vi "KlingerV2 GetAxisParams.vi"(0 "Axe":u8(ring) items=["W", "X", "Y", "Z"], 5 "Param":T1, 11 "error in":errorcluster) -> (1 "ID Number":i32, 2 "Speed":cluster{"Vitesse":i32, "Accel":dbl}={"Vitesse"=800, "Accel"=0.4000000059604645} {"Accel" min=0.10000000149011612 max=2.0 step=0.10000000149011612 format="%#.1f"; "Vitesse" min=32 max=4000 step=1 format="%#.0f"}, 3 "TypeMouv":i32(ring) caption="Type de mouvement" items=["Linéaire", "Rotation"], 4 "Nom de l'axe":string, 6 "Type":i32(ring) caption="Type de moteur" items=["UE30", "UE72"], 8 "FactConv":dbl=0.01 caption="Facteur de\nConversion\n(m/pas ou °/pas)", 10 "CorrParams":T2={"CorrActive"=FALSE, "ErreurLim"=0.1, "NbrEssais"=3} caption="Paramètres de correction de position" {"NbrEssais" min=1 max=5 step=1; "ErreurLim" min=0.0 max=10.0 step=0.1 format="%#.1f"}, 13 "Encodeur":bool caption="Possède un\nEncodeur", 14 "Origine":bool caption="Possède un\nInterrupteur d'origine", 15 "error out":errorcluster)   [LabVIEW 2010]
doc: "Ce Vi lit les paramètres des différents axes moteur, qui sont enregistrer dans un fichier .ini."
uses:
  <userlib>/KlingerV2/KlingerV2 Params.ctl
  <vilib>/Utility/config.llb/Read Key (I32).vi
  <vilib>/Utility/config.llb/Read Key (Double).vi
  <vilib>/Utility/config.llb/Read Key (Boolean).vi
  <vilib>/Utility/config.llb/Read Key (String).vi
  <vilib>/Utility/config.llb/NI_LVConfig.lvlib
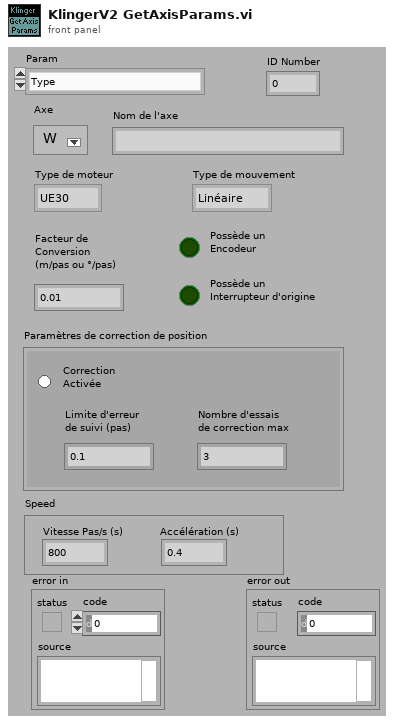
[diagram p1: front panel]
types:
  T1 = typedef "KlingerV2 Params.ctl" = enum16{"Type", "Origine", "Encodeur", "TypeMouv", "FactConv", "Nom", "CorrParams", "KlingCtrlPar", "Speed", "Acc", "Avance", "Tous"}
  T2 = cluster{"CorrActive":bool, "ErreurLim":dbl, "NbrEssais":i32}
  T3 = typedef "NI_LVConfig.lvlib/Config Data RefNum.ctl" = refnum<k1>
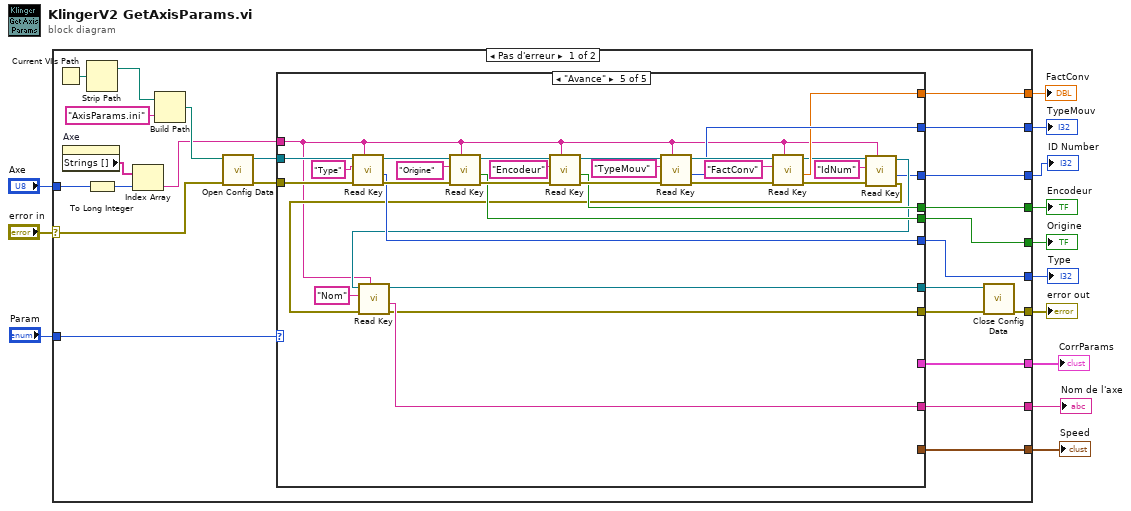
[diagram p0: block diagram]
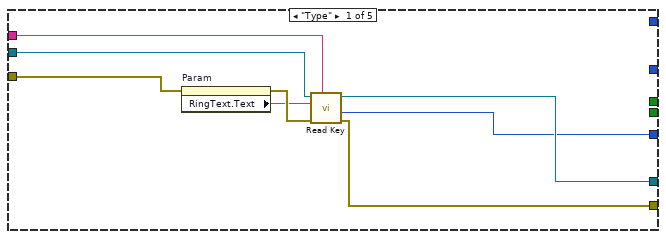
[diagram p2: hidden frame]
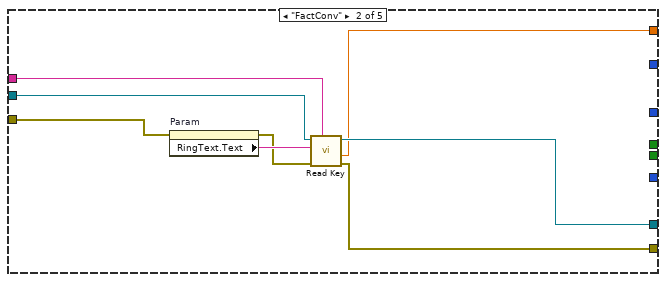
[diagram p3: hidden frame]
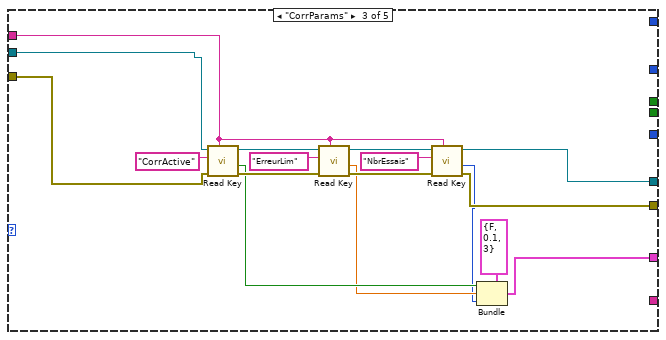
[diagram p4: hidden frame]
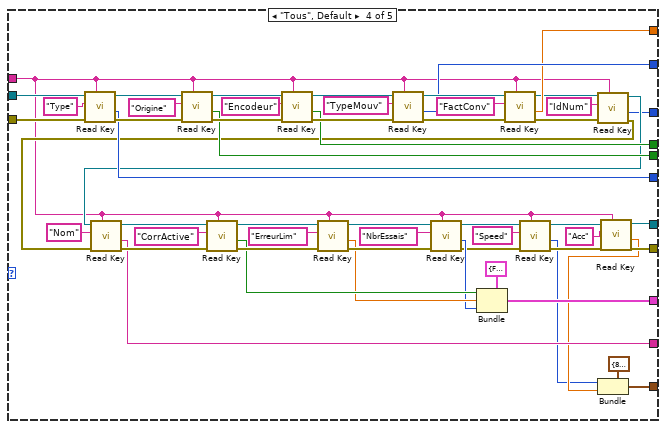
[diagram p5: hidden frame]
diagram:
  n1 = case shown="Pas d'erreur" "error in" {
    selector: "error in" -> [w34 w156]
    tunnel: "Axe" -> [w33 _]
    tunnel: [w26 w156] -> w12
    tunnel: [w23 _] -> w10
    tunnel: [w22 _] -> w9
    tunnel: [w21 _] -> w8
    tunnel: [w20 _] -> w7
    tunnel: [w19 _] -> w6
    tunnel: [w18 _] -> w5
    tunnel: [w17 _] -> w4
    tunnel: "Param" -> [w16 _]
    tunnel: [w15 _] -> w2
    tunnel: [w14 _] -> w1
    frame No Error {
      n2 = Current VI's Path() -> (path=w37:path)
      n3 = property on="Axe" class="MDér (strict)"() -> ("Strings []"=w31:string[])  [unwired: 2 in, 2 out]
      n4 = Strip Path(path=w37) -> (stripped path=w24:path)  [unwired: 1 out]
      n5 = To Long Integer(number=w33) -> (32bit integer=w32:i32)
      n6 = Index Array(array=w31, index=w32) -> (element=w25:string)
      n7 = Build Path(base path=w24, name or relative path="AxisParams.ini") -> (appended path=w35:path)
      n8 = call <vilib>:"Open Config Data.vi"("error in (no error)"=w34, "configuration file path"=w35) -> ("error out"=w29:errorcluster, "refnum"=w30:T3)  [unwired: 7 in, 1 out]
      n9 = case shown="\"Avance\"" w16 {
        tunnel: w30 -> [w45 w53 w61 w116 w150]
        tunnel: w29 -> [w40 w47 w59 w115 w149]
        tunnel: [w42 w50 w60 w84 w126] -> w28
        tunnel: [w43 w51 w63 w87 w125] -> w27
        tunnel: w25 -> [w44 w52 w62 w71 w127]
        tunnel: [_ w49 _ w77 w133] -> w23
        tunnel: [_ _ _ w95 w139] -> w22
        tunnel: [_ _ _ w94 w138] -> w21
        tunnel: [_ _ _ w93 w137] -> w20
        tunnel: [w41 _ _ w92 w136] -> w19
        tunnel: [_ _ w54 w91 _] -> w18
        tunnel: [_ _ _ w90 w135] -> w17
        tunnel: [_ _ _ w79 _] -> w15
        tunnel: [_ _ _ w72 w128] -> w14
        frame "Type" {
          n10 = property on="Param" class="Énum (strict)"(error in=w40) -> (error out=w39:errorcluster, "RingText.Text"=w38:string)  [unwired: 1 in, 1 out]
          n11 = call-poly <vilib>:"Read Key.vi"("section"=w44, "error in (no error)"=w39, "key"=w38, "refnum"=w45) -> ("error out"=w43:errorcluster, "value"=w41:i32, "refnum out"=w42:T3)  [unwired: 4 in, 1 out]
        }
        frame "FactConv" {
          n12 = property on="Param" class="Énum (strict)"(error in=w47) -> (error out=w46:errorcluster, "RingText.Text"=w48:string)  [unwired: 1 in, 1 out]
          n13 = call-poly <vilib>:"Read Key.vi"("section"=w52, "error in (no error)"=w46, "key"=w48, "refnum"=w53) -> ("error out"=w51:errorcluster, "value"=w49:dbl, "refnum out"=w50:T3)  [unwired: 4 in, 1 out]
        }
        frame "CorrParams" {
          n14 = call-poly <vilib>:"Read Key.vi"("section"=w62, "error in (no error)"=w59, "key"="CorrActive", "refnum"=w61) -> ("error out"=w66:errorcluster, "value"=w57:bool, "refnum out"=w67:T3)  [unwired: 4 in, 1 out]
          n15 = call-poly <vilib>:"Read Key.vi"("section"=w62, "error in (no error)"=w66, "key"="ErreurLim", "refnum"=w67) -> ("error out"=w64:errorcluster, "value"=w56:dbl, "refnum out"=w65:T3)  [unwired: 4 in, 1 out]
          n16 = call-poly <vilib>:"Read Key.vi"("section"=w62, "error in (no error)"=w64, "key"="NbrEssais", "refnum"=w65) -> ("error out"=w63:errorcluster, "value"=w55:i32, "refnum out"=w60:T3)  [unwired: 4 in, 1 out]
          n17 = Bundle(cluster=T2 {"CorrActive"=FALSE, "ErreurLim"=0.1, "NbrEssais"=3} ("CorrParams"), "CorrActive"=w57, "ErreurLim"=w56, "NbrEssais"=w55) -> (w54:T2)
        }
        frame "Tous", Default {
          n18 = call-poly <vilib>:"Read Key.vi"("section"=w71, "error in (no error)"=w115, "key"="Type", "refnum"=w116) -> ("error out"=w112:errorcluster, "value"=w92:i32, "refnum out"=w114:T3)  [unwired: 4 in, 1 out]
          n19 = call-poly <vilib>:"Read Key.vi"("section"=w71, "error in (no error)"=w112, "key"="Origine", "refnum"=w114) -> ("error out"=w111:errorcluster, "value"=w93:bool, "refnum out"=w106:T3)  [unwired: 4 in, 1 out]
          n20 = call-poly <vilib>:"Read Key.vi"("section"=w71, "error in (no error)"=w111, "key"="Encodeur", "refnum"=w106) -> ("error out"=w110:errorcluster, "value"=w94:bool, "refnum out"=w107:T3)  [unwired: 4 in, 1 out]
          n21 = call-poly <vilib>:"Read Key.vi"("section"=w71, "error in (no error)"=w110, "key"="TypeMouv", "refnum"=w107) -> ("error out"=w109:errorcluster, "value"=w95:i32, "refnum out"=w108:T3)  [unwired: 4 in, 1 out]
          n22 = call-poly <vilib>:"Read Key.vi"("section"=w71, "error in (no error)"=w109, "key"="FactConv", "refnum"=w108) -> ("error out"=w78:errorcluster, "value"=w77:dbl, "refnum out"=w76:T3)  [unwired: 4 in, 1 out]
          n23 = call-poly <vilib>:"Read Key.vi"("section"=w71, "error in (no error)"=w78, "key"="IdNum", "refnum"=w76) -> ("error out"=w74:errorcluster, "value"=w72:i32, "refnum out"=w75:T3)  [unwired: 4 in, 1 out]
          n24 = call-poly <vilib>:"Read Key.vi"("section"=w71, "error in (no error)"=w74, "key"="Nom", "refnum"=w75) -> ("error out"=w104:errorcluster, "value"=w90:string, "refnum out"=w105:T3)  [unwired: 4 in, 1 out]
          n25 = call-poly <vilib>:"Read Key.vi"("section"=w71, "error in (no error)"=w104, "key"="CorrActive", "refnum"=w105) -> ("error out"=w102:errorcluster, "value"=w98:bool, "refnum out"=w103:T3)  [unwired: 4 in, 1 out]
          n26 = call-poly <vilib>:"Read Key.vi"("section"=w71, "error in (no error)"=w102, "key"="ErreurLim", "refnum"=w103) -> ("error out"=w100:errorcluster, "value"=w97:dbl, "refnum out"=w101:T3)  [unwired: 4 in, 1 out]
          n27 = call-poly <vilib>:"Read Key.vi"("section"=w71, "error in (no error)"=w100, "key"="NbrEssais", "refnum"=w101) -> ("error out"=w88:errorcluster, "value"=w96:i32, "refnum out"=w89:T3)  [unwired: 4 in, 1 out]
          n28 = Bundle(cluster=T2 {"CorrActive"=FALSE, "ErreurLim"=0.1, "NbrEssais"=3} ("CorrParams"), "CorrActive"=w98, "ErreurLim"=w97, "NbrEssais"=w96) -> (w91:T2)
          n29 = call-poly <vilib>:"Read Key.vi"("section"=w71, "error in (no error)"=w88, "key"="Speed", "refnum"=w89) -> ("error out"=w87:errorcluster, "value"=w80:i32, "refnum out"=w85:T3)  [unwired: 4 in, 1 out]
          n30 = call-poly <vilib>:"Read Key.vi"("section"=w71, "key"="Acc", "refnum"=w85) -> ("value"=w81:dbl, "refnum out"=w84:T3)  [unwired: 5 in, 2 out]
          n31 = Bundle(cluster=cluster{"Vitesse":i32, "Accel":dbl} {"Vitesse"=800, "Accel"=0.4000000059604645} ("Speed"), "Vitesse"=w80, "Accel"=w81) -> (w79:cluster{"Vitesse":i32, "Accel":dbl})
        }
        frame "Avance" {
          n32 = call-poly <vilib>:"Read Key.vi"("section"=w127, "error in (no error)"=w149, "key"="Type", "refnum"=w150) -> ("error out"=w146:errorcluster, "value"=w136:i32, "refnum out"=w148:T3)  [unwired: 4 in, 1 out]
          n33 = call-poly <vilib>:"Read Key.vi"("section"=w127, "error in (no error)"=w146, "key"="Origine", "refnum"=w148) -> ("error out"=w145:errorcluster, "value"=w137:bool, "refnum out"=w140:T3)  [unwired: 4 in, 1 out]
          n34 = call-poly <vilib>:"Read Key.vi"("section"=w127, "error in (no error)"=w145, "key"="Encodeur", "refnum"=w140) -> ("error out"=w144:errorcluster, "value"=w138:bool, "refnum out"=w141:T3)  [unwired: 4 in, 1 out]
          n35 = call-poly <vilib>:"Read Key.vi"("section"=w127, "error in (no error)"=w144, "key"="TypeMouv", "refnum"=w141) -> ("error out"=w143:errorcluster, "value"=w139:i32, "refnum out"=w142:T3)  [unwired: 4 in, 1 out]
          n36 = call-poly <vilib>:"Read Key.vi"("section"=w127, "error in (no error)"=w143, "key"="FactConv", "refnum"=w142) -> ("error out"=w134:errorcluster, "value"=w133:dbl, "refnum out"=w132:T3)  [unwired: 4 in, 1 out]
          n37 = call-poly <vilib>:"Read Key.vi"("section"=w127, "error in (no error)"=w134, "key"="IdNum", "refnum"=w132) -> ("error out"=w130:errorcluster, "value"=w128:i32, "refnum out"=w131:T3)  [unwired: 4 in, 1 out]
          n38 = call-poly <vilib>:"Read Key.vi"("section"=w127, "error in (no error)"=w130, "key"="Nom", "refnum"=w131) -> ("error out"=w125:errorcluster, "value"=w135:string, "refnum out"=w126:T3)  [unwired: 4 in, 1 out]
        }
      }
      n39 = call <vilib>:"Close Config Data.vi"("error in (no error)"=w27, "refnum"=w28) -> ("error out"=w26:errorcluster)  [unwired: 8 in, 1 out]
    }
    frame Error {
    }
  }
  "error out" <- w12
  "TypeMouv" <- w9
  "FactConv" <- w10
  "Encodeur" <- w8
  "Origine" <- w7
  "Type" <- w6
  "CorrParams" <- w5
  "Nom de l'axe" <- w4
  "Speed" <- w2
  "ID Number" <- w1
